vi "AAA Charger_Catalog, Mid-Level.vi"   [LabVIEW 2010]
uses:
  Charger_Status Refnum.ctl
panel:
  # "Charger Catalog"
types:
  T1 = typedef "Charger_Status Refnum.ctl" = refnum<vi>
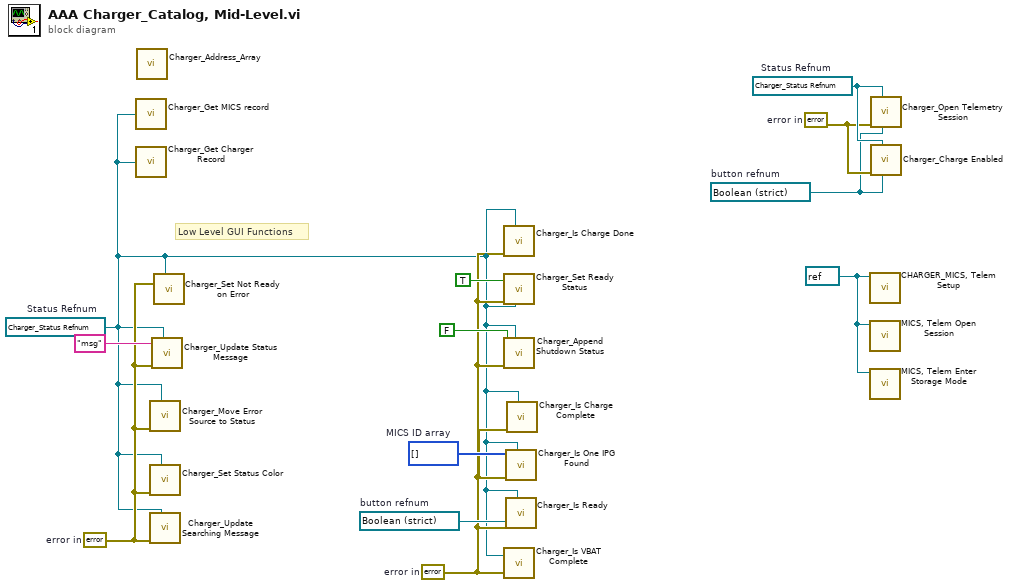
[diagram p0: block diagram]
diagram:
  w4 = refnum<vi> refnum  # button refnum
  w6 = T1 refnum  # Status Refnum
  w5 = errorcluster {"status"=FALSE, "code"=0, "source"=""}  # error in
  w10 = u32[] []  # MICS ID array
  w11 = refnum<vi> refnum  # button refnum
  w1 = T1 refnum  # Status Refnum
  w2 = errorcluster {"status"=FALSE, "code"=0, "source"=""}  # error in
  w8 = refnum<visa-resource-name> refnum ("VISA Resource")
  w3 = errorcluster {"status"=FALSE, "code"=0, "source"=""}  # error in
  # "Low Level GUI Functions"
  n1 = call "Charger_Get MICS record.vi"("Status Refnum"=w1) -> ()  [unwired: 4 in, 5 out]
  n2 = call "Charger_Get Charger Record.vi"("Status Refnum"=w1) -> ()  [unwired: 4 in, 5 out]
  n3 = call "Charger_Address_Array.vi"() -> ()  [unwired: 7 in, 3 out]
  n4 = call "Charger_Move Error Source to Status.vi"("error in"=w2, "Status Refnum"=w1) -> ()  [unwired: 8 in, 1 out]
  n5 = call "Charger_Set Status Color.vi"("error in"=w2, "Status Refnum"=w1) -> ()  [unwired: 8 in, 1 out]
  n6 = call "Charger_Update Searching Message.vi"("Status Refnum"=w1, "error in"=w2) -> ()  [unwired: 7 in, 1 out]
  n7 = call "Charger_Update Status Message.vi"("Status Refnum"=w1, "error in"=w2, "status message"="msg") -> ()  [unwired: 6 in, 1 out]
  n8 = call "Charger_Set Not Ready on Error.vi"("Status Refnum"=w1, "error in"=w2) -> ()  [unwired: 7 in, 2 out]
  n9 = call "Charger_Is Charge Done.vi"("Status Refnum"=w1, "error in"=w3) -> ()  [unwired: 8 in, 2 out]
  n10 = call "Charger_Set Ready Status.vi"("Ready"=TRUE, "Status Refnum"=w1, "error in"=w3) -> ()  [unwired: 6 in, 2 out]
  n11 = call "Charger_Append Shutdown Status.vi"("Status Refnum"=w1, "error in"=w3, "Base Station Idle"=FALSE ("idle")) -> ()  [unwired: 6 in, 1 out]
  n12 = call "Charger_Is VBAT Complete.vi"("Status Refnum"=w1, "error in"=w3) -> ()  [unwired: 8 in, 2 out]
  n13 = call "Charger_Is One IPG Found.vi"("Status Refnum"=w1, "error in"=w3, "MICS ID array"=w10) -> ()  [unwired: 4 in, 3 out]
  n14 = call "Charger_Is Ready.vi"("Stop Refnum"=w11, "Status Refnum"=w1, "error in"=w3) -> ()  [unwired: 7 in, 2 out]
  n15 = call "Charger_Is Charge Complete.vi"("Status Refnum"=w1, "error in"=w3) -> ()  [unwired: 8 in, 2 out]
  n16 = call "CHARGER_MICS, Telem Setup.vi"("VISA resource"=w8) -> ()  [unwired: 9 in, 2 out]
  n17 = call "MICS, Telem Open Session.vi"("VISA resource"=w8) -> ()  [unwired: 8 in, 3 out]
  n18 = call "MICS, Telem Enter Storage Mode.vi"("VISA resource"=w8) -> ()  [unwired: 9 in, 2 out]
  n19 = call "Charger_Open Telemetry Session.vi"("Stop Refnum"=w4, "Status Refnum"=w6, "error in"=w5) -> ()  [unwired: 7 in, 2 out]
  n20 = call "Charger_Charge Enabled.vi"("Stop Refnum"=w4, "Status Refnum"=w6, "error in"=w5) -> ()  [unwired: 8 in, 1 out]
